vi "Test.vi"() -> ()   [LabVIEW 2017, in "Performance.lvlib"]
uses:
  Performance.lvlib
panel:
  out "Memory Usage (%)":dbl
  out "CPU Usage (%)":dbl
  out "Chart":cluster{"CPU Usage":dbl, "Memory Available":dbl}(graph)
  in  "Stop":bool
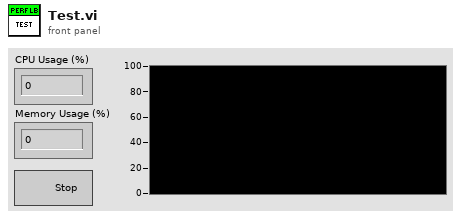
[diagram p1: front panel]
types:
  T1 = typedef "Performance.lvlib/Performance Data.ctl" = cluster{"CPU Usage (%)":dbl, "Memory Usage (%)":dbl, "CPU Usage Ref":T2, "Initialized":bool}
  T2 = typedef "Performance.lvlib/tools_system CPU Usage Ref.ctl" = cluster{"Query":u32, "Counter":u32}
  T3 = cluster{"CPU Usage (%)":dbl, "Memory Usage (%)":dbl}
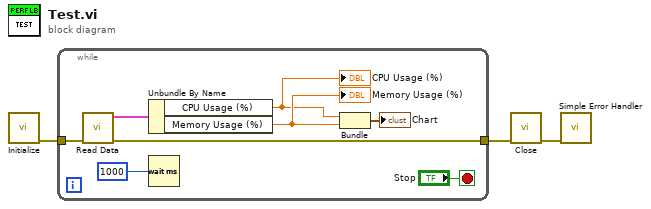
[diagram p0: block diagram]
diagram:
  n1 = call "Initialize.vi"() -> ("error out"=w3:errorcluster)  [unwired: 11 in]
  n2 = while {
    tunnel: w3 -> [w11]
    tunnel: [w10] -> w2
    stop <- "Stop" stop-if-true
    n3 = call "Read Data.vi"("error in (no error)"=w11) -> ("error out"=w10:errorcluster, "Performance Data"=w7:T1)  [unwired: 9 in]
    n4 = Unbundle By Name(w7) -> ("CPU Usage (%)"=w4:dbl, "Memory Usage (%)"=w6:dbl)
    "CPU Usage (%)" <- w4
    "Memory Usage (%)" <- w6
    n5 = Wait (ms)(milliseconds to wait=u32 1000) -> ()  [unwired: 1 out]
    n6 = Bundle("CPU Usage (%)"=w4, "Memory Usage (%)"=w6) -> (→"Chart":T3)  [unwired: 1 in]
  }
  n7 = call "Close.vi"("error in (no error)"=w2) -> ("error out"=w1:errorcluster)  [unwired: 10 in]
  n8 = call <vilib>:"Simple Error Handler.vi"("error in (no error)"=w1) -> ()  [unwired: 4 in, 5 out]
